vi "PLL analyzer -- PID -- V3.vi"(0 "frequency IN (Hz)":dbl=-1.0 format="%#_10f", 1 "voltage IN (V)":cdb=-0.0017981943418797428+0.0018232090265536353i format="%#_10f", 4 "time in (sec)":dbl=289.5873590533738, 5 "lorentzian IN":T5={"A (VHz)"=0.003914650866681924, "ω (Hz)"=44855.11779996251, "Γ (Hz)"=2.9247633391664567, "φ (rad)"=3.909694945239435, "Q"=15336.32386569301, "Norm  Ampl"=nan, "z∞ (V)"=0.00013625172364348747-0.00019483842623467182i, "4corners"={"z (-pi/2)"=-0.0017563199699203156-0.00016210148449623068i, "z(inf)"=0.00013625172364348747-0.00019483842623467182i, "z (pi/2)"=0.0001689886653819286+0.0016977332673291314i, "z center"=-0.0007936656522691936+0.0007678158914164503i, "z(0)"=-0.0017235830281818747+0.0017304702090675725i, "radius"=0.0013384504702515796}} {"z∞ (V)" format="%#_4p"; "Q" format="%#_4p"; "φ (rad)" format="%#_3p"; "Γ (Hz)" format="%#_5p"; "ω (Hz)" format="%#_9p"; "A (VHz)" format="%#_3p"}, 6 "PID action":T7, 7 "requested size":i32=100, 9 "OWL parameters":T1={"T (sec)"=1.2701010101010102, "owl?"=enum."focus", "A (rad)"=1.2701010101010102, "refit ?"=enum."refit"} {"T (sec)" scale=1.0..20.0; "A (rad)" scale=0.1..1.57}, 10 "PLL limits (Hz)":dbl=5000.0 format="%#.2f", 11 "PID mode":T4, 12 "dt (sec)":dbl=0.02 format="%#_10f", 13 "PID parameters":T8={"I (sec)"=4.747474747474747, "P (sec)"=2.0765656565656565} {"P (sec)" scale=0.01..10.0 scale format="%#_2p"; "I (sec)" scale=0.01..10.0 scale format="%#_2p"}) -> (14 "frequency OUT (Hz)":dbl=-1.0 format="%#_10f", 15 "overlimit ?":bool=TRUE, 17 "phase OUT (rad)":dbl=-1.0 format="%#_10f", 18 "time out (sec)":dbl=289.5873590533738, 19 "lorentzian  OUT":T5={"A (VHz)"=0.003914650866681924, "ω (Hz)"=44855.11779996251, "Γ (Hz)"=2.9247633391664567, "φ (rad)"=3.909694945239435, "Q"=15336.32386569301, "Norm  Ampl"=nan, "z∞ (V)"=0.00013625172364348747-0.00019483842623467182i, "4corners"={"z (-pi/2)"=-0.0017563199699203156-0.00016210148449623068i, "z(inf)"=0.00013625172364348747-0.00019483842623467182i, "z (pi/2)"=0.0001689886653819286+0.0016977332673291314i, "z center"=-0.0007936656522691936+0.0007678158914164503i, "z(0)"=-0.0017235830281818747+0.0017304702090675725i, "radius"=0.0013384504702515796}} {"z∞ (V)" format="%#_4p"; "Q" format="%#_4p"; "φ (rad)" format="%#_3p"; "Γ (Hz)" format="%#_5p"; "ω (Hz)" format="%#_9p"; "A (VHz)" format="%#_3p"})   [LabVIEW 2021]
uses:
  pid -- parameters.ctl
  PID action.ctl
  lorentzian.ctl
  circle corners.ctl
  PID - mode.ctl
  owl parameters.ctl
  owl action.ctl
  owl -- send for fit action.ctl
  agregator -- action.ctl
  four-corner circle transformation.ctl
  Q - not nan -- real.vi
  linear interpolation iiii- complex.vi
  linear interpolation - real.vi
panel:
  out "voltage OUT (V)":cdb=-0.0017981943418797428+0.0018232090265536353i format="%#_10f"
  out "Plot: complex plane":cluster{dbl[], dbl[]}[](graph)=[{[], []}, {[nan, nan, nan, nan, nan, nan, nan, nan, nan, nan, nan, nan, nan, nan, nan, nan, nan, nan, nan, nan, nan, nan, nan, nan, nan, nan, nan, nan, nan, nan, nan, nan, nan, nan, nan, nan, nan, nan, nan, nan, nan, nan, nan, nan, nan, nan, nan, nan, nan, nan], [nan, nan, nan, nan, nan, nan, nan, nan, nan, nan, nan, nan, nan, nan, nan, nan, nan, nan, nan, nan, nan, nan, nan, nan, nan, nan, nan, nan, nan, nan, nan, nan, nan, nan, nan, nan, nan, nan, nan, nan, nan, nan, nan, nan, nan, nan, nan, nan, nan, nan]}, {[nan, nan, nan, nan, nan, nan, nan, nan, nan, nan, nan, nan, nan, nan, nan, nan, nan, nan, nan, nan], [nan, nan, nan, nan, nan, nan, nan, nan, nan, nan, nan, nan, nan, nan, nan, nan, nan, nan, nan, nan]}, {[nan, nan, nan, nan, nan, nan, nan, nan, nan, nan, nan, nan, nan, nan, nan, nan, nan, nan, nan, nan], [nan, nan, nan, nan, nan, nan, nan, nan, nan, nan, nan, nan, nan, nan, nan, nan, nan, nan, nan, nan]}, {[nan, nan, nan, nan, nan, nan, nan, nan, nan, nan, nan, nan, nan, nan, nan, nan, nan, nan, nan, nan], [nan, nan, nan, nan, nan, nan, nan, nan, nan, nan, nan, nan, nan, nan, nan, nan, nan, nan, nan, nan]}, {[nan, nan, nan, nan, nan, nan, nan, nan, nan, nan, nan, nan, nan, nan, nan, nan, nan, nan, nan, nan], [nan, nan, nan, nan, nan, nan, nan, nan, nan, nan, nan, nan, nan, nan, nan, nan, nan, nan, nan, nan]}, {[], []}]
  in  "Plot: complex plane - filter":cluster{dbl[], dbl[]}[](graph)=[{[], []}, {[], []}, {[0.0, 0.0, 0.0, 0.0, 0.0, 0.0, 0.0, 0.0, 0.0, 0.0, 0.0, 0.0, 0.0, 0.0, 0.0, 0.0, 0.0, 0.0, 0.0, 0.0, 0.0, 0.0, 0.0, 0.0, 0.0, 0.0, 0.0, 0.0, 0.0, 0.0, 0.0, 0.0, 0.0, 0.0, 0.0, 0.0, 0.0, 0.0, 0.0, 0.0, 0.0, 0.0, 0.0, 0.0, 0.0, 0.0, 0.0, 0.0, 0.0, 0.0, 0.0, 0.0, 0.0, 0.0, 0.0, 0.0, 0.0, 0.0, 0.0, 0.0, 0.0, 0.0, 0.0, 0.0, 0.0, 0.0, 0.0, 0.0, 0.0, 0.0, 0.0, 0.0, 0.0, 0.0, 0.0, 0.0, 0.0, 0.0, 0.0, 0.0, 0.0, 0.0, 0.0, 0.0, 0.0, 0.0, 0.0, 0.0, 0.0, 0.0, 0.0, 0.0, 0.0, 0.0, 0.0, 0.0, 0.0, 0.0, 0.0, 0.0], [0.0, 0.0, 0.0, 0.0, 0.0, 0.0, 0.0, 0.0, 0.0, 0.0, 0.0, 0.0, 0.0, 0.0, 0.0, 0.0, 0.0, 0.0, 0.0, 0.0, 0.0, 0.0, 0.0, 0.0, 0.0, 0.0, 0.0, 0.0, 0.0, 0.0, 0.0, 0.0, 0.0, 0.0, 0.0, 0.0, 0.0, 0.0, 0.0, 0.0, 0.0, 0.0, 0.0, 0.0, 0.0, 0.0, 0.0, 0.0, 0.0, 0.0, 0.0, 0.0, 0.0, 0.0, 0.0, 0.0, 0.0, 0.0, 0.0, 0.0, 0.0, 0.0, 0.0, 0.0, 0.0, 0.0, 0.0, 0.0, 0.0, 0.0, 0.0, 0.0, 0.0, 0.0, 0.0, 0.0, 0.0, 0.0, 0.0, 0.0, 0.0, 0.0, 0.0, 0.0, 0.0, 0.0, 0.0, 0.0, 0.0, 0.0, 0.0, 0.0, 0.0, 0.0, 0.0, 0.0, 0.0, 0.0, 0.0, 0.0]}, {[0.0, 0.0, 0.0], [0.0, 0.0, 0.0]}, {[nan, nan, nan, nan, nan, nan, nan, nan, nan, nan, nan, nan, nan, nan, nan, nan, nan, nan, nan, nan], [nan, nan, nan, nan, nan, nan, nan, nan, nan, nan, nan, nan, nan, nan, nan, nan, nan, nan, nan, nan]}, {[0.0, 0.0, 0.0, 0.0, 0.0, 0.0, 0.0, 0.0, 0.0, 0.0, 0.0, 0.0, 0.0, 0.0, 0.0, 0.0, 0.0, 0.0, 0.0, 0.0], [0.0, 0.0, 0.0, 0.0, 0.0, 0.0, 0.0, 0.0, 0.0, 0.0, 0.0, 0.0, 0.0, 0.0, 0.0, 0.0, 0.0, 0.0, 0.0, 0.0]}]
  out "pm lorentzian":T5={"A (VHz)"=nan, "ω (Hz)"=0.0, "Γ (Hz)"=0.0, "φ (rad)"=nan, "Q"=nan, "Norm  Ampl"=nan, "z∞ (V)"=nan+nani, "4corners"={"z (-pi/2)"=nan+nani, "z(inf)"=nan+nani, "z (pi/2)"=nan+nani, "z center"=nan+nani, "z(0)"=nan+nani, "radius"=nan}} {"z∞ (V)" format="%#_4p"; "Q" format="%#_4p"; "φ (rad)" format="%#_3p"; "Γ (Hz)" format="%#_5p"; "ω (Hz)" format="%#_9p"; "A (VHz)" format="%#_3p"}
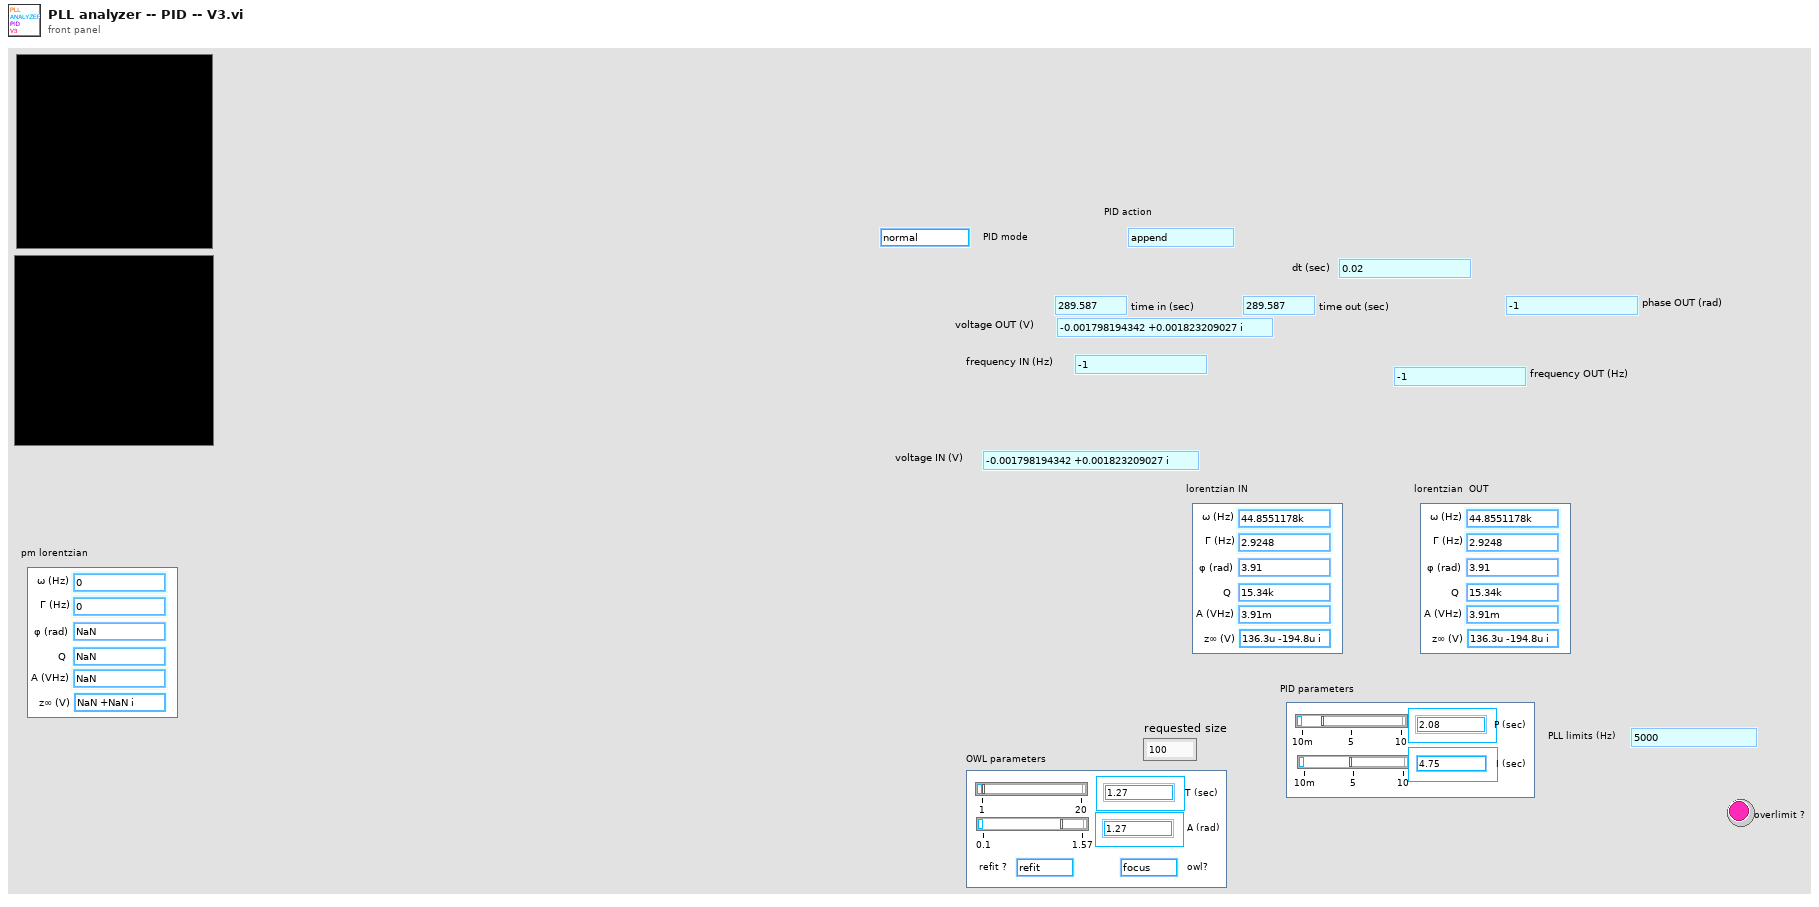
[diagram p1: front panel]
types:
  T1 = typedef "owl parameters.ctl" = cluster{"T (sec)":dbl, "owl?":T2, "A (rad)":dbl, "refit ?":T3}
  T2 = typedef "owl action.ctl" = enum16{"owl", "focus"}
  T3 = typedef "owl -- send for fit action.ctl" = enum16{"refit", "chill"}
  T4 = typedef "PID - mode.ctl" = enum16{"normal", "heat"}
  T5 = typedef "lorentzian.ctl" = cluster{"A (VHz)":dbl, "ω (Hz)":dbl, "Γ (Hz)":dbl, "φ (rad)":dbl, "Q":dbl, "Norm  Ampl":dbl, "z∞ (V)":cdb, "4corners":T6}
  T6 = typedef "circle corners.ctl" = cluster{"z (-pi/2)":cdb, "z(inf)":cdb, "z (pi/2)":cdb, "z center":cdb, "z(0)":cdb, "radius":dbl}
  T7 = typedef "PID action.ctl" = enum16{"append", "empty!", "reset frequency", "reset from num", "overlimit"}
  T8 = typedef "pid -- parameters.ctl" = cluster{"I (sec)":dbl, "P (sec)":dbl}
  T9 = typedef "agregator -- action.ctl" = enum16{"append", "interpolate", "empty!", "force", "init", "scale", "read last"}
  T10 = typedef "four-corner circle transformation.ctl" = enum16{"z(c) z(inf)", "z(c) z(zero)", "fix phase", "calculate lorentzian", "z(0) z(+-pi/2)", "shift to zcenter", "to  canonical", "get canonical phase", "get4corners", "update lorentzian -- from z0", "fake gamma normal", "fake gamma heat", "calculate complex slope", "get f0 given f and phi"}
  T11 = typedef "interpolation state - real.ctl" = cluster{"Array ":dbl[], "actual size":i32, "requested size":i32}
  T12 = typedef "interpolation state - complex.ctl" = cluster{"requested size":i32, "Array":cdb[], "actual number of elements":i32}
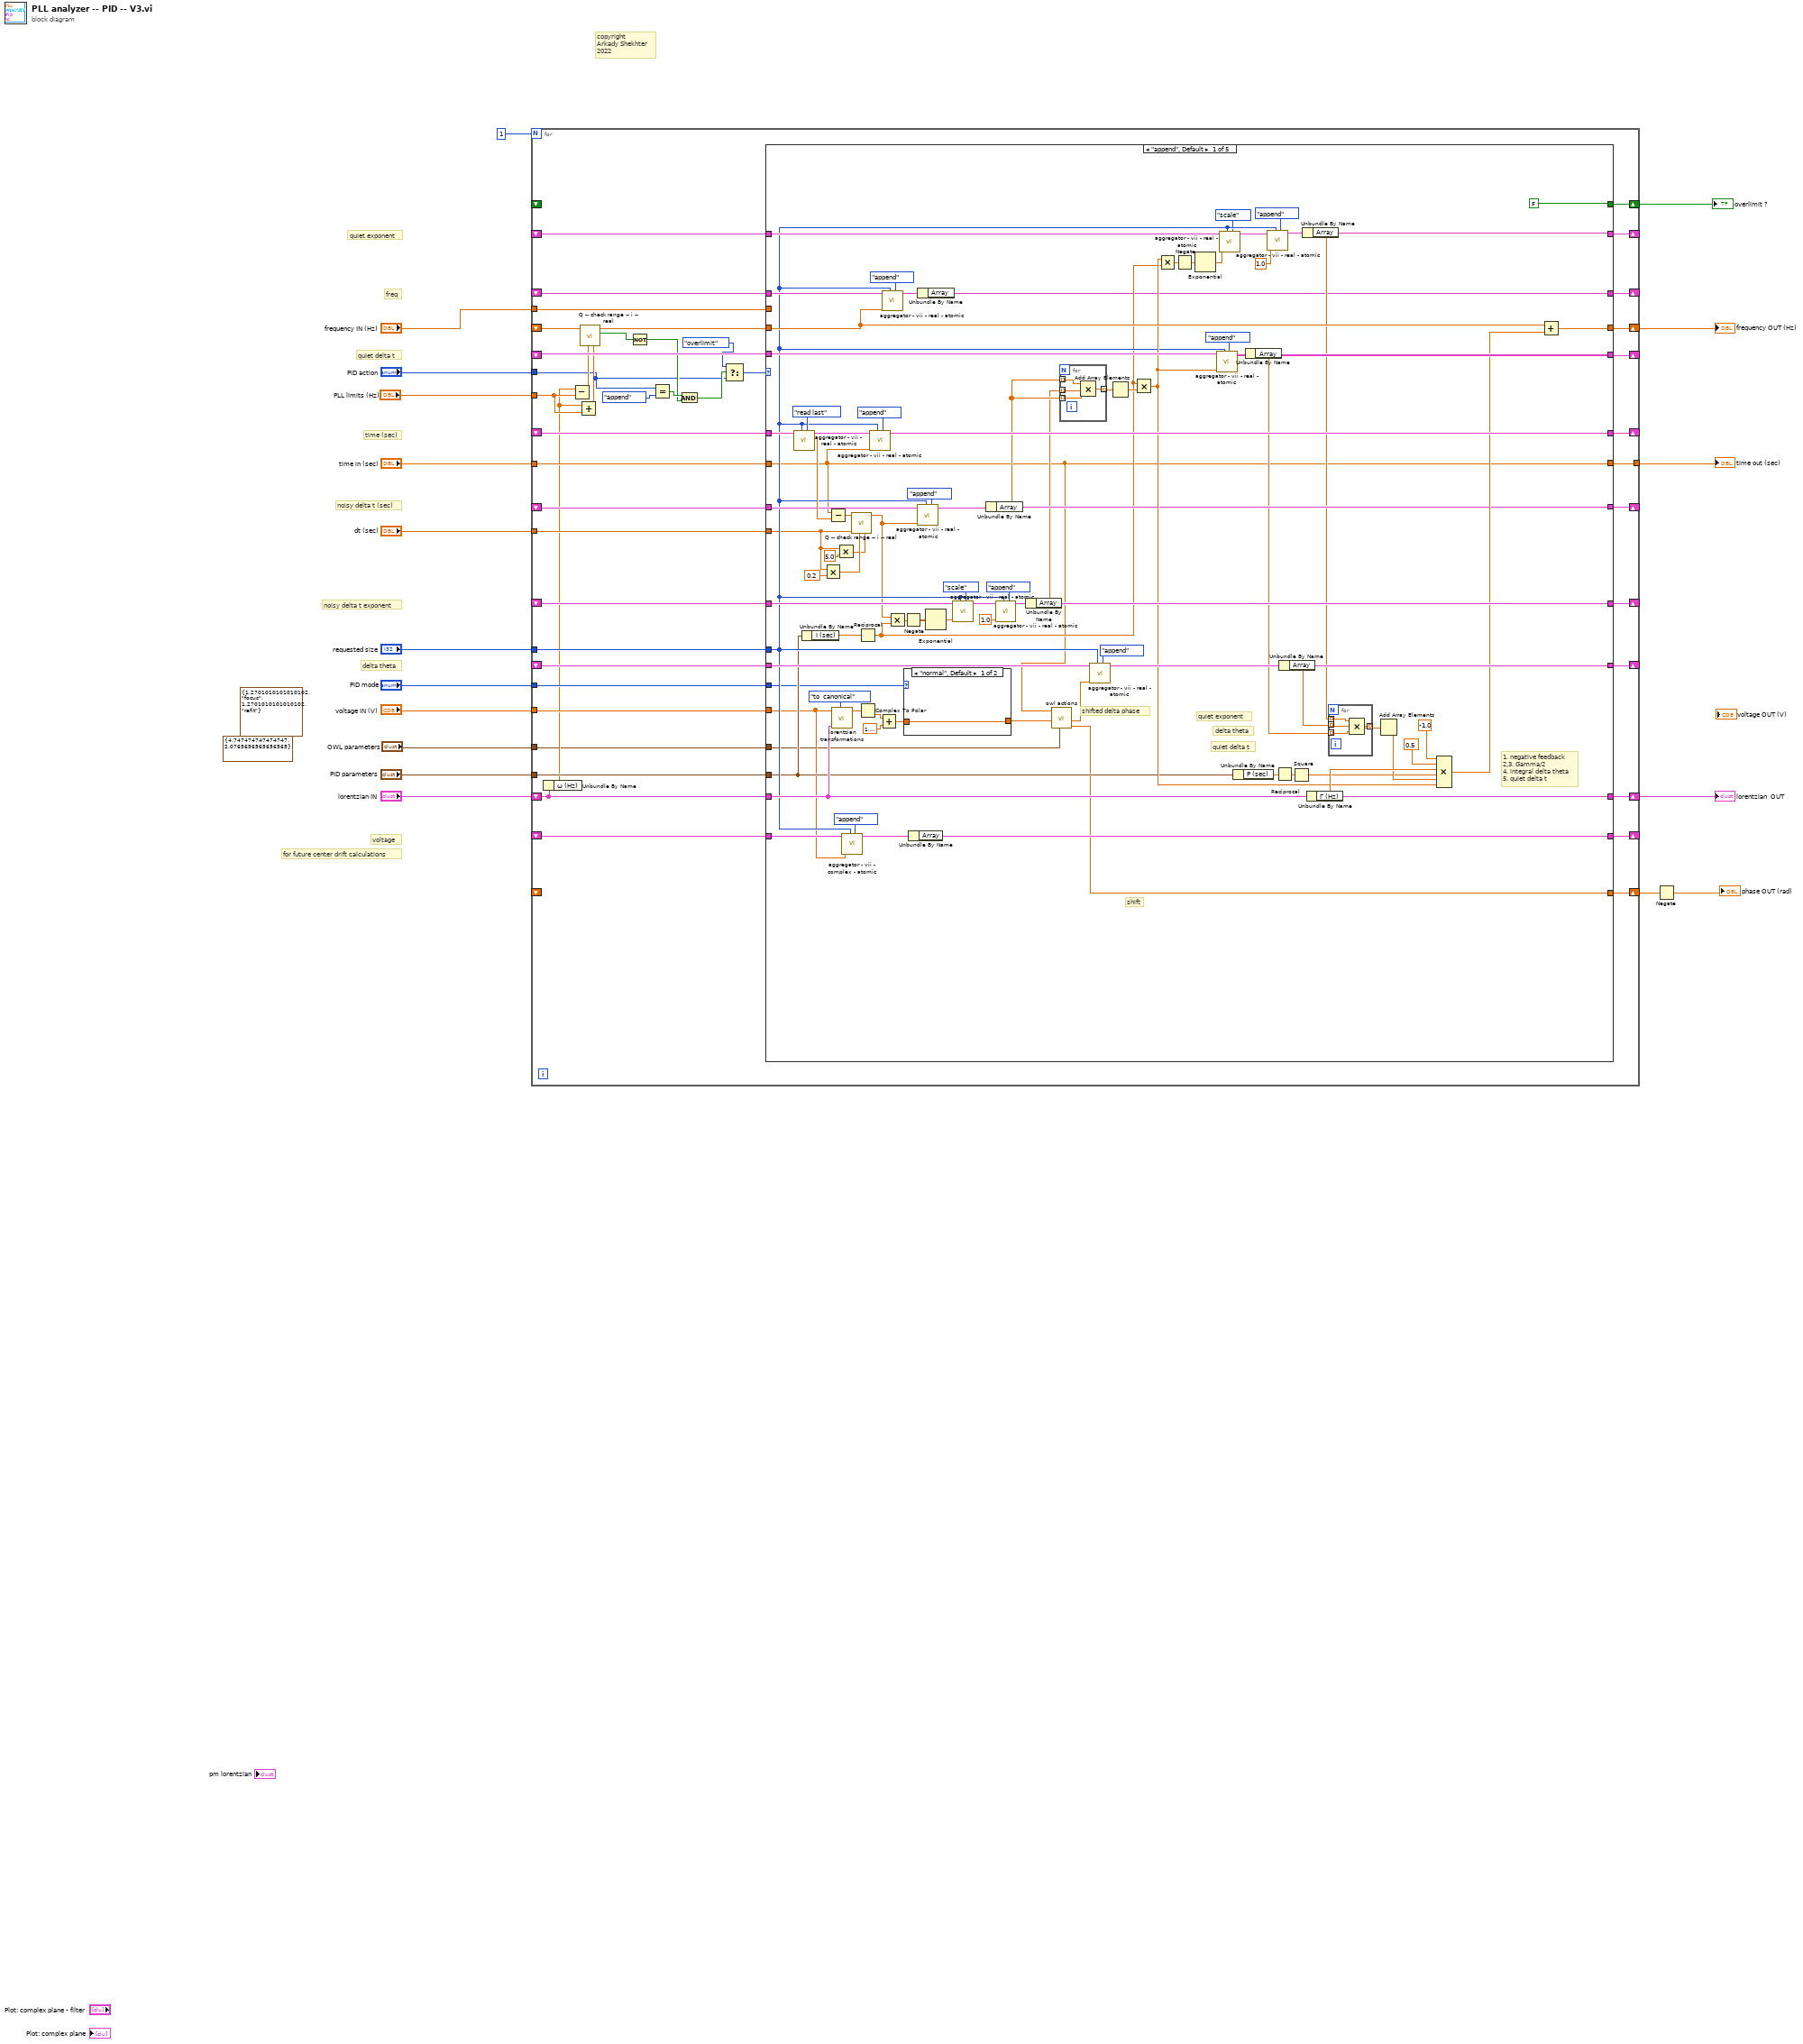
[diagram p0: block diagram]
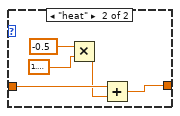
[diagram p2: hidden frame]
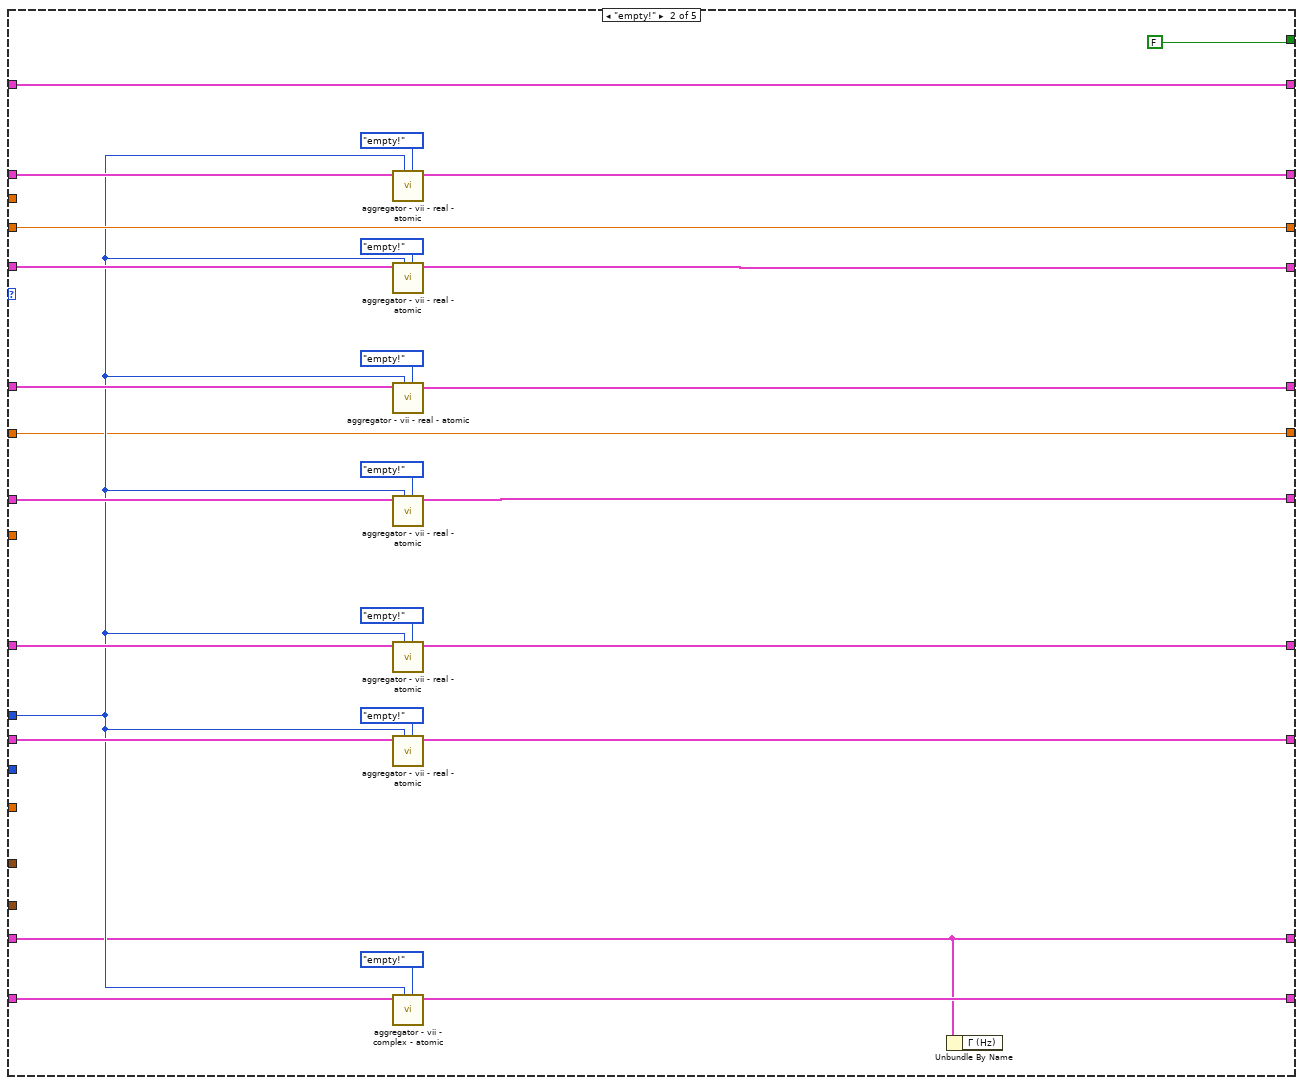
[diagram p3: hidden frame]
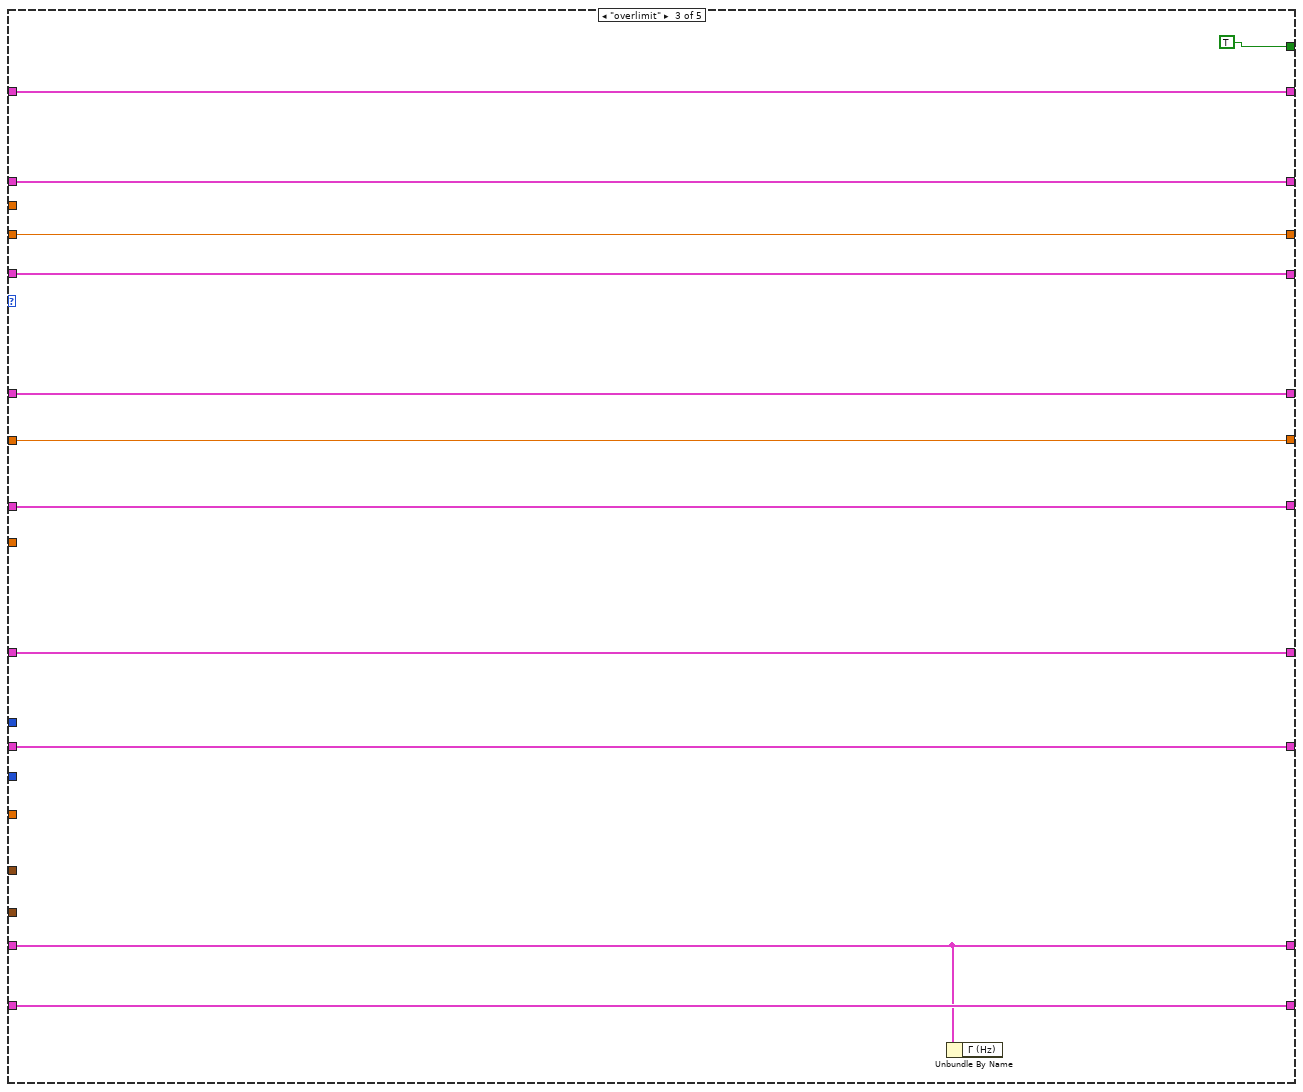
[diagram p4: hidden frame]
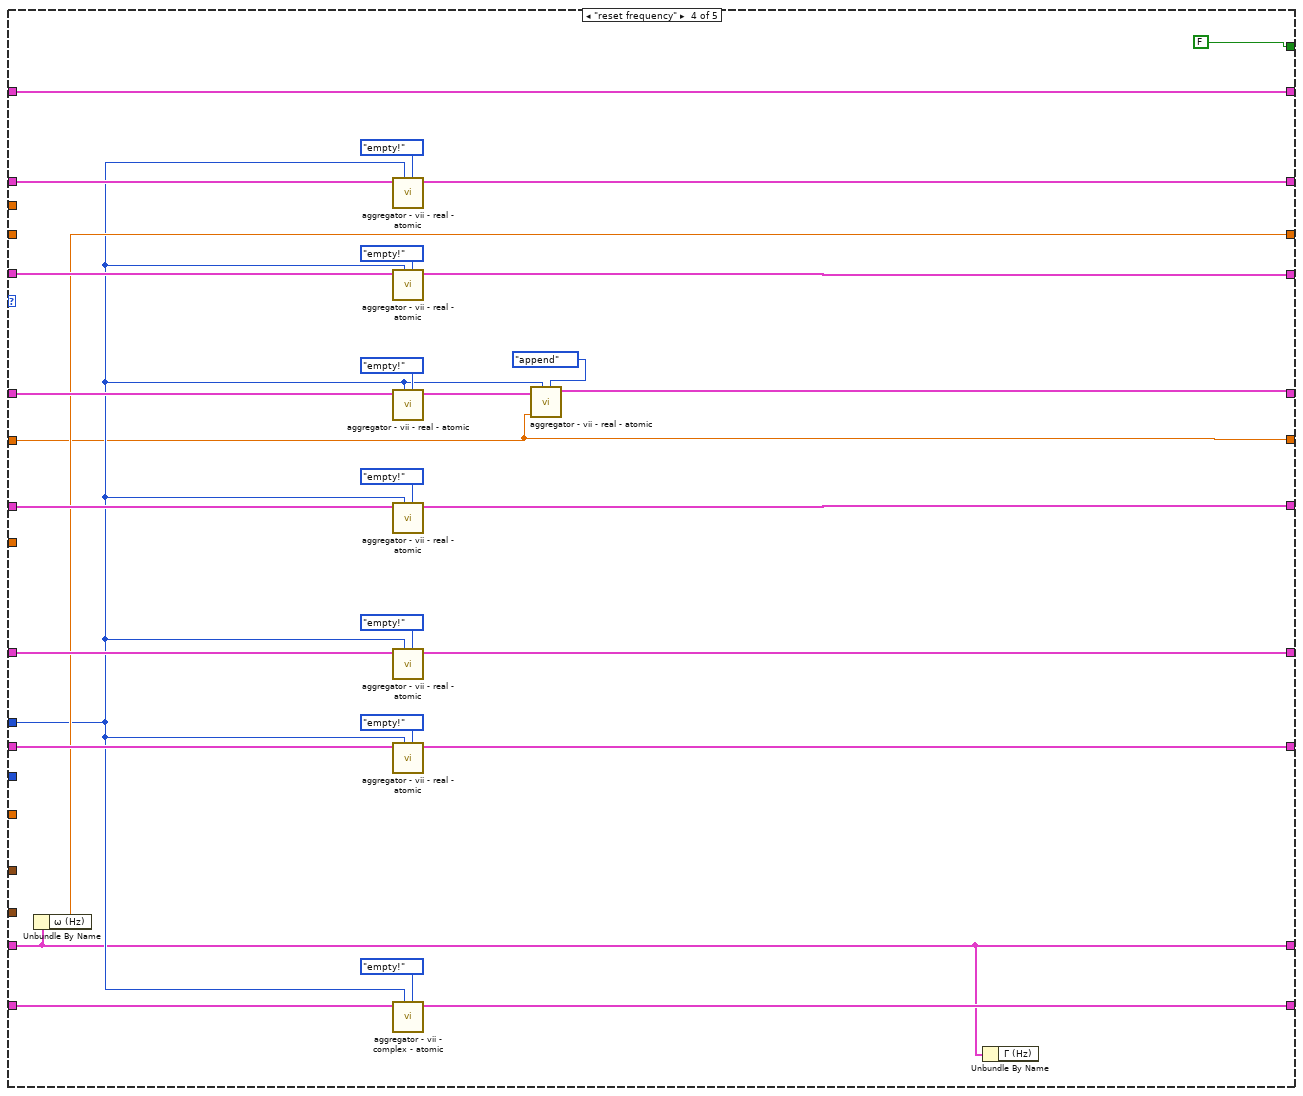
[diagram p5: hidden frame]
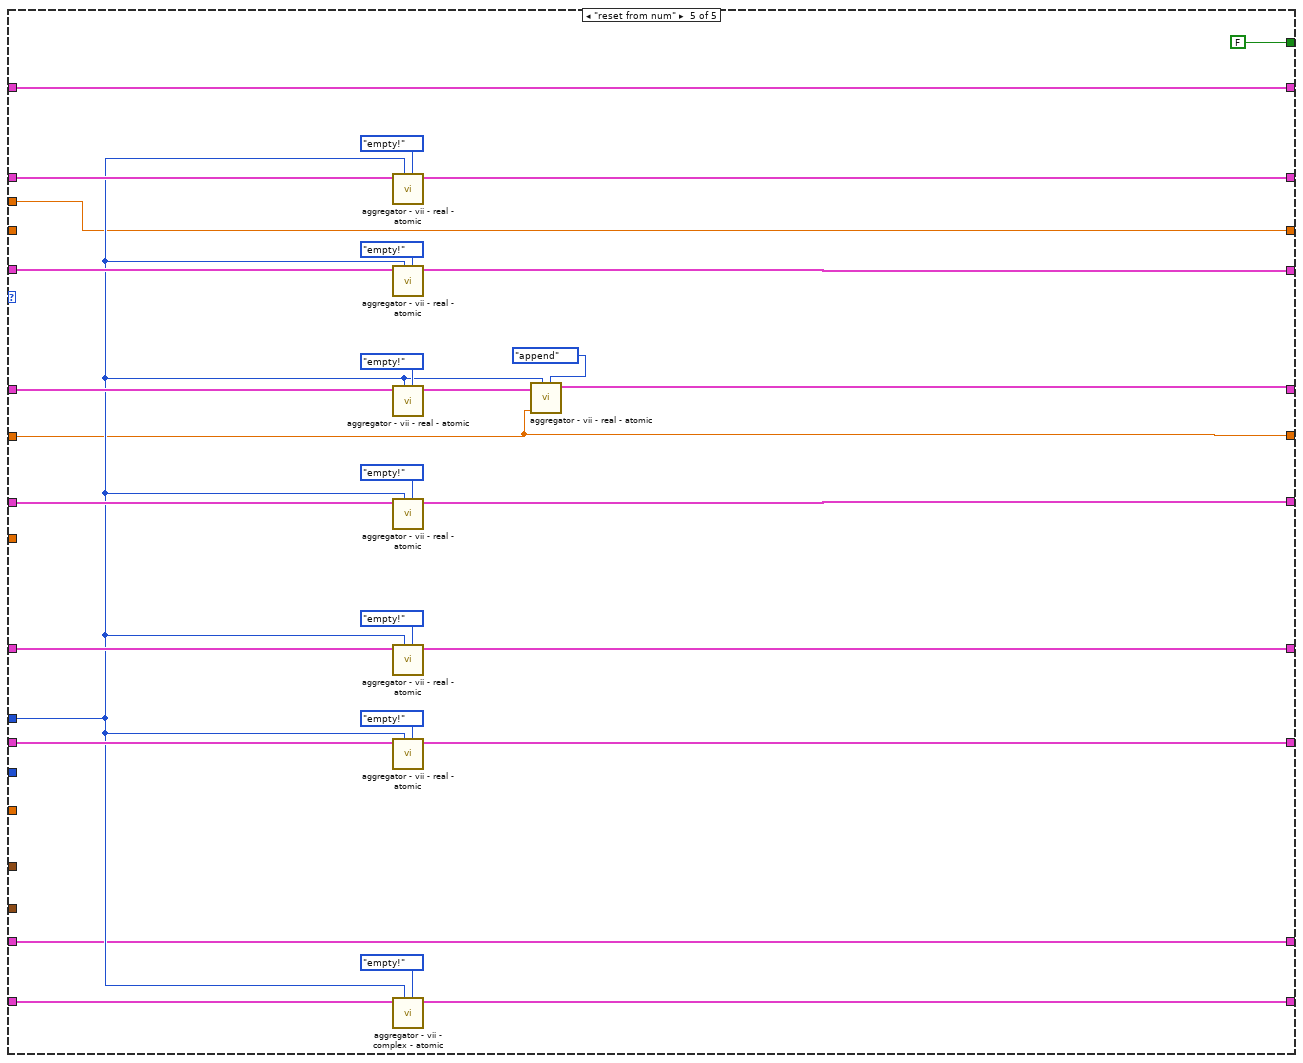
[diagram p6: hidden frame]
diagram:
  (unwired) T8 {"I (sec)"=4.747474747474747, "P (sec)"=2.0765656565656565} ("PID parameters")
  (unwired) T1 {"T (sec)"=1.2701010101010102, "owl?"=enum."focus", "A (rad)"=1.2701010101010102, "refit ?"=enum."refit"} ("OWL parameters")
  # "copyright\nArkady Shekhter\n2022"
  # "quiet exponent"
  # "noisy delta t exponent"
  # "for future center drift calculations"
  # "voltage"
  # "freq"
  # "delta theta"
  # "quiet delta t"
  # "time (sec)"
  # "noisy delta t (sec)"
  n1 = for {
    N: 1 -> [_]
    tunnel: "requested size" -> [w62]
    tunnel: "PID action" -> [w21]
    shift-right: [w60] -> _
    shift-left: _ -> [w61]
    tunnel: "time in (sec)" -> [w59]
    shift-right: [w57] -> _
    shift-left: _ -> [w58]
    tunnel: "voltage IN (V)" -> [w56]
    shift-right: [w54] -> _
    shift-left: _ -> [w55]
    shift-right: [w52] -> _
    shift-left: _ -> [w53]
    shift-right: [w51] -> w7
    shift-left: _ -> [w31]
    shift-right: [w50] -> w13
    shift-left: "lorentzian IN" -> [w33]
    shift-right: [w49] -> _
    shift-left: _ -> [w48]
    shift-right: [w47] -> _
    shift-left: _ -> [w46]
    shift-right: [w45] -> _
    shift-left: _ -> [w44]
    shift-right: [w43] -> _
    shift-left: _ -> [w42]
    tunnel: "frequency IN (Hz)" -> [w41]
    tunnel: "dt (sec)" -> [w40]
    tunnel: "PID parameters" -> [w39]
    tunnel: [w38] -> w9
    tunnel: "PID mode" -> [w37]
    tunnel: "PLL limits (Hz)" -> [w34]
    shift-right: [w28] -> w5
    shift-left: _ -> [_]
    tunnel: "OWL parameters" -> [w20]
    shift-right: [w19] -> w2
    shift-left: _ -> [_]
    n2 = Unbundle By Name(w33) -> ("ω (Hz)"=w32:dbl)
    n3 = Subtract(x=w32, y=w34) -> (x-y=w36:dbl)
    n4 = Add(x=w32, y=w34) -> (x+y=w35:dbl)
    n5 = call "Q -- check range -- i -- real.vi"("upper"=w35, "lower"=w36, "number"=w31) -> ("in range?"=w25:bool, "number in range"=w30:dbl)  [unwired: 6 in, 1 out]
    n6 = Not(x=w25) -> (.not. x?=w24:bool)
    n7 = Equal?(x=w21, y=PID_action."append" ("f")) -> (x = y?=w26:bool)
    n8 = And(x=w26, y=w24) -> (x .and. y?=w23:bool)
    n9 = Select(t=PID_action."overlimit" ("f"), s=w23, f=w21) -> (s? t:f=w29:T7)
    n10 = case shown="\"append\", Default" w29 {
      tunnel: w62 -> [w103 w164 _ w203 w233]
      tunnel: w61 -> [w145 w176 w195 w217 w246]
      tunnel: [w126 w163 w195 w204 w234] -> w60
      tunnel: w59 -> [w65 w162 w189 w202 w232]
      tunnel: w58 -> [w144 w180 w197 w221 w250]
      tunnel: [w131 w179 w197 w220 w249] -> w57
      tunnel: w56 -> [w72 _ _ _ _]
      tunnel: w55 -> [w111 w178 w196 w219 w248]
      tunnel: [w98 w177 w196 w218 w247] -> w54
      tunnel: w53 -> [w135 w182 w198 w223 w252]
      tunnel: [w133 w181 w198 w222 w251] -> w52
      tunnel: w30 -> [w116 w175 w194 _ _]
      tunnel: w33 -> [w119 w161 w188 w199 w228]
      tunnel: [w128 w175 w194 w207 w230] -> w51
      tunnel: [w119 w161 w188 w199 w228] -> w50
      tunnel: [w69 w173 w193 w201 w231] -> w49
      tunnel: w48 -> [w118 w174 w193 w216 w245]
      tunnel: [w68 w169 w192 w212 w241] -> w47
      tunnel: w46 -> [w117 w170 w192 w213 w242]
      tunnel: [w100 w167 w191 w210 w239] -> w45
      tunnel: w44 -> [w108 w166 w191 w209 w238]
      tunnel: [w99 w165 w190 w208 w237] -> w43
      tunnel: w42 -> [w107 w165 w190 w208 w237]
      tunnel: w41 -> [_ _ _ _ w230]
      tunnel: w40 -> [w83 _ _ _ _]
      tunnel: w39 -> [w76 _ _ _ _]
      tunnel: [w65 w162 w189 w202 w232] -> w38
      tunnel: w37 -> [w71 _ _ _ _]
      tunnel: [FALSE FALSE TRUE FALSE FALSE] -> w28
      tunnel: w20 -> [w67 _ _ _ _]
      tunnel: [w63 _ _ _ _] -> w19
      frame "append", Default {
        # "shift"
        # "shifted delta phase"
        # "1. negative feedback\n2,3. Gamma/2\n4. integral delta theta\n5. quiet delta t"
        # "quiet delta t"
        # "delta theta"
        # "quiet exponent"
        n11 = call "aggregator - vii - real - atomic.vi"("aggregator action"=agregator_--_action."read last", "requested size"=w103, "state IN"=w145) -> ("mean"=w138:dbl, "state OUT"=w127:T11)  [unwired: 5 in, 2 out]
        n12 = Unbundle By Name(w76) -> ("I (sec)"=w75:dbl)
        n13 = Multiply(x=w83, y=0.2 ("upper")) -> (x*y=w89:dbl)
        n14 = Subtract(x=w65, y=w138) -> (x-y=w93:dbl)
        n15 = call "lorentzian transformations.vi"("4 corner circle transformation"=four-corner_circle_transformation."to  canonical", "lorentzian in"=w119, "voltage in"=w72) -> ("voltage out"=w123:cdb)  [unwired: 5 in, 3 out]
        n16 = Multiply(x=w83, y=5.0 ("upper")) -> (x*y=w81:dbl)
        n17 = call "aggregator - vii - complex - atomic.vi"("aggregator action"=agregator_--_action."append", "requested size"=w103, "number"=w72, "state IN"=w118) -> ("state OUT"=w69:T12)  [unwired: 4 in, 3 out]
        n18 = call "Q -- check range -- i -- real.vi"("upper"=w81, "lower"=w89, "default"=w83, "number"=w93) -> ("number in range"=w91:dbl)  [unwired: 5 in, 2 out]
        n19 = Reciprocal(x=w75) -> (1/x=w74:dbl)
        n20 = Complex To Polar(r * e^(i*theta)=w123) -> (theta=w122:dbl)  [unwired: 1 out]
        n21 = call "aggregator - vii - real - atomic.vi"("aggregator action"=agregator_--_action."append", "requested size"=w103, "number"=w65, "state IN"=w127) -> ("state OUT"=w126:T11)  [unwired: 4 in, 3 out]
        n22 = Add(x=w122, y=1.5707963267948966) -> (x+y=w73:dbl)
        n23 = call "aggregator - vii - real - atomic.vi"("aggregator action"=agregator_--_action."append", "requested size"=w103, "number"=w116, "state IN"=w117) -> ("state OUT"=w68:T11)  [unwired: 4 in, 3 out]
        n24 = Multiply(x=w91, y=w74) -> (x*y=w95:dbl)
        n25 = Negate(x=w95) -> (-x=w92:dbl)
        n26 = case shown="\"normal\", Default" w71 {
          tunnel: w73 -> [w146 w151]
          tunnel: [w146 w150] -> w66
          frame "normal", Default {
          }
          frame "heat" {
            n27 = Multiply(x=-0.5, y=1.5707963267948966) -> (x*y=w147:dbl)
            n28 = Add(x=w151, y=w147) -> (x+y=w150:dbl)
          }
        }
        n29 = Unbundle By Name(w69) -> ()  [unwired: 1 out]
        n30 = Unbundle By Name(w68) -> ()  [unwired: 1 out]
        n31 = call "aggregator - vii - real - atomic.vi"("aggregator action"=agregator_--_action."append", "requested size"=w103, "number"=w91, "state IN"=w111) -> ("state OUT"=w98:T11)  [unwired: 4 in, 3 out]
        n32 = Exponential(1:w92) -> (0:w94:dbl)
        n33 = call "aggregator - vii - real - atomic.vi"("aggregator action"=agregator_--_action."scale", "requested size"=w103, "number"=w94, "state IN"=w144) -> ("state OUT"=w143:T11)  [unwired: 4 in, 3 out]
        n34 = Unbundle By Name(w98) -> ("Array"=w110:dbl[])
        n35 = call "aggregator - vii - real - atomic.vi"("aggregator action"=agregator_--_action."append", "requested size"=w103, "number"=1.0, "state IN"=w143) -> ("state OUT"=w131:T11)  [unwired: 4 in, 3 out]
        n36 = Unbundle By Name(w131) -> ("Array"=w97:dbl[])
        n37 = call "owl actions.vi"("OWL parameters"=w67, "delta phase (rad) IN"=w66, "time in (sec)"=w65) -> ("phase (rad) OUT"=w63:dbl, "delta phase (rad) OUT"=w64:dbl)  [unwired: 7 in]
        n38 = for {
          tunnel: [w155] -> w112 mode=indexing
          tunnel: w110 -> [w154] mode=indexing
          tunnel: w97 -> [w153] mode=indexing
          tunnel: w110 -> [w152] mode=indexing
          n39 = Compound Arithmetic op=MULTIPLY(w154, w153, w152) -> (w155:dbl)
        }
        n40 = call "aggregator - vii - real - atomic.vi"("aggregator action"=agregator_--_action."append", "requested size"=w103, "number"=w64, "state IN"=w135) -> ("state OUT"=w133:T11)  [unwired: 4 in, 3 out]
        n41 = Add Array Elements(numeric array=w112) -> (sum=w82:dbl)
        n42 = Multiply(x=w74, y=w82) -> (x*y=w106:dbl)
        n43 = Multiply(x=w106, y=w74) -> (x*y=w86:dbl)
        n44 = Negate(x=w86) -> (-x=w85:dbl)
        n45 = Exponential(1:w85) -> (0:w84:dbl)
        n46 = call "aggregator - vii - real - atomic.vi"("aggregator action"=agregator_--_action."append", "requested size"=w103, "number"=w106, "state IN"=w108) -> ("state OUT"=w100:T11)  [unwired: 4 in, 3 out]
        n47 = call "aggregator - vii - real - atomic.vi"("aggregator action"=agregator_--_action."scale", "requested size"=w103, "number"=w84, "state IN"=w107) -> ("state OUT"=w105:T11)  [unwired: 4 in, 3 out]
        n48 = Unbundle By Name(w76) -> ("P (sec)"=w79:dbl)
        n49 = Unbundle By Name(w100) -> ("Array"=w88:dbl[])
        n50 = call "aggregator - vii - real - atomic.vi"("aggregator action"=agregator_--_action."append", "requested size"=w103, "number"=1.0, "state IN"=w105) -> ("state OUT"=w99:T11)  [unwired: 4 in, 3 out]
        n51 = Reciprocal(x=w79) -> (1/x=w78:dbl)
        n52 = Unbundle By Name(w133) -> ("Array"=w96:dbl[])
        n53 = Square(x=w78) -> (x^2=w77:dbl)
        n54 = Unbundle By Name(w99) -> ("Array"=w87:dbl[])
        n55 = Unbundle By Name(w119) -> ("Γ (Hz)"=w130:dbl)
        n56 = for {
          tunnel: w96 -> [w159] mode=indexing
          tunnel: [w158] -> w132 mode=indexing
          tunnel: w88 -> [w157] mode=indexing
          tunnel: w87 -> [w156] mode=indexing
          n57 = Compound Arithmetic op=MULTIPLY(w156, w159, w157) -> (w158:dbl)
        }
        n58 = Add Array Elements(numeric array=w132) -> (sum=w129:dbl)
        n59 = Compound Arithmetic op=MULTIPLY(-1.0 ("value"), 0.5 ("value"), w130, w77, w129, w106) -> (w113:dbl)
        n60 = Add(x=w116, y=w113) -> (x+y=w128:dbl)
      }
      frame "empty!" {
        n61 = call "aggregator - vii - real - atomic.vi"("aggregator action"=agregator_--_action."empty!", "requested size"=w164, "state IN"=w170) -> ("state OUT"=w169:T11)  [unwired: 5 in, 3 out]
        n62 = call "aggregator - vii - real - atomic.vi"("aggregator action"=agregator_--_action."empty!", "requested size"=w164, "state IN"=w166) -> ("state OUT"=w167:T11)  [unwired: 5 in, 3 out]
        n63 = call "aggregator - vii - real - atomic.vi"("aggregator action"=agregator_--_action."empty!", "requested size"=w164, "state IN"=w176) -> ("state OUT"=w163:T11)  [unwired: 5 in, 3 out]
        n64 = call "aggregator - vii - real - atomic.vi"("aggregator action"=agregator_--_action."empty!", "requested size"=w164, "state IN"=w178) -> ("state OUT"=w177:T11)  [unwired: 5 in, 3 out]
        n65 = call "aggregator - vii - real - atomic.vi"("aggregator action"=agregator_--_action."empty!", "requested size"=w164, "state IN"=w180) -> ("state OUT"=w179:T11)  [unwired: 5 in, 3 out]
        n66 = call "aggregator - vii - real - atomic.vi"("aggregator action"=agregator_--_action."empty!", "requested size"=w164, "state IN"=w182) -> ("state OUT"=w181:T11)  [unwired: 5 in, 3 out]
        n67 = call "aggregator - vii - complex - atomic.vi"("aggregator action"=agregator_--_action."empty!", "requested size"=w164, "state IN"=w174) -> ("state OUT"=w173:T12)  [unwired: 5 in, 3 out]
        n68 = Unbundle By Name(w161) -> ()  [unwired: 1 out]
      }
      frame "overlimit" {
        n69 = Unbundle By Name(w188) -> ()  [unwired: 1 out]
      }
      frame "reset frequency" {
        n70 = Unbundle By Name(w199) -> ("ω (Hz)"=w207:dbl)
        n71 = call "aggregator - vii - real - atomic.vi"("aggregator action"=agregator_--_action."empty!", "requested size"=w203, "state IN"=w213) -> ("state OUT"=w212:T11)  [unwired: 5 in, 3 out]
        n72 = call "aggregator - vii - real - atomic.vi"("aggregator action"=agregator_--_action."empty!", "requested size"=w203, "state IN"=w209) -> ("state OUT"=w210:T11)  [unwired: 5 in, 3 out]
        n73 = call "aggregator - vii - real - atomic.vi"("aggregator action"=agregator_--_action."empty!", "requested size"=w203, "state IN"=w217) -> ("state OUT"=w205:T11)  [unwired: 5 in, 3 out]
        n74 = call "aggregator - vii - real - atomic.vi"("aggregator action"=agregator_--_action."empty!", "requested size"=w203, "state IN"=w219) -> ("state OUT"=w218:T11)  [unwired: 5 in, 3 out]
        n75 = call "aggregator - vii - real - atomic.vi"("aggregator action"=agregator_--_action."empty!", "requested size"=w203, "state IN"=w221) -> ("state OUT"=w220:T11)  [unwired: 5 in, 3 out]
        n76 = call "aggregator - vii - real - atomic.vi"("aggregator action"=agregator_--_action."empty!", "requested size"=w203, "state IN"=w223) -> ("state OUT"=w222:T11)  [unwired: 5 in, 3 out]
        n77 = call "aggregator - vii - complex - atomic.vi"("aggregator action"=agregator_--_action."empty!", "requested size"=w203, "state IN"=w216) -> ("state OUT"=w201:T12)  [unwired: 5 in, 3 out]
        n78 = call "aggregator - vii - real - atomic.vi"("aggregator action"=agregator_--_action."append", "requested size"=w203, "number"=w202, "state IN"=w205) -> ("state OUT"=w204:T11)  [unwired: 4 in, 3 out]
        n79 = Unbundle By Name(w199) -> ()  [unwired: 1 out]
      }
      frame "reset from num" {
        n80 = call "aggregator - vii - real - atomic.vi"("aggregator action"=agregator_--_action."empty!", "requested size"=w233, "state IN"=w242) -> ("state OUT"=w241:T11)  [unwired: 5 in, 3 out]
        n81 = call "aggregator - vii - real - atomic.vi"("aggregator action"=agregator_--_action."empty!", "requested size"=w233, "state IN"=w238) -> ("state OUT"=w239:T11)  [unwired: 5 in, 3 out]
        n82 = call "aggregator - vii - real - atomic.vi"("aggregator action"=agregator_--_action."empty!", "requested size"=w233, "state IN"=w246) -> ("state OUT"=w235:T11)  [unwired: 5 in, 3 out]
        n83 = call "aggregator - vii - real - atomic.vi"("aggregator action"=agregator_--_action."empty!", "requested size"=w233, "state IN"=w248) -> ("state OUT"=w247:T11)  [unwired: 5 in, 3 out]
        n84 = call "aggregator - vii - real - atomic.vi"("aggregator action"=agregator_--_action."empty!", "requested size"=w233, "state IN"=w250) -> ("state OUT"=w249:T11)  [unwired: 5 in, 3 out]
        n85 = call "aggregator - vii - real - atomic.vi"("aggregator action"=agregator_--_action."empty!", "requested size"=w233, "state IN"=w252) -> ("state OUT"=w251:T11)  [unwired: 5 in, 3 out]
        n86 = call "aggregator - vii - complex - atomic.vi"("aggregator action"=agregator_--_action."empty!", "requested size"=w233, "state IN"=w245) -> ("state OUT"=w231:T12)  [unwired: 5 in, 3 out]
        n87 = call "aggregator - vii - real - atomic.vi"("aggregator action"=agregator_--_action."append", "requested size"=w233, "number"=w232, "state IN"=w235) -> ("state OUT"=w234:T11)  [unwired: 4 in, 3 out]
      }
    }
  }
  "lorentzian  OUT" <- w13
  "time out (sec)" <- w9
  "frequency OUT (Hz)" <- w7
  "overlimit ?" <- w5
  n88 = Negate(x=w2) -> (-x=→"phase OUT (rad)":dbl)
